vi "RG Configure DAQ auto Max input scale.vi"(4 "input terminal configuration":i32(ring)=10106 items=["default"=-1, "RSE"=10083, "NRSE"=10078, "Differential"=10106, "Pseudodifferential"=12529], 6 "DAQ Card Type":enum16{"USB-6211", "USB-6251", "USB-6361"}(ring)=enum."USB-6251", 7 "Sampling rate":dbl=20000.0, 8 "error in":errorcluster, 9 "DAQ Trigger Level":dbl format="%0.2f", 10 "physical channel":string="Dev2/ai0", 11 "number of samples":i32=100000) -> (0 "error out":errorcluster, 3 "task out":refnum<k21>)   [LabVIEW 2017, in "DAQ.lvlib"]
uses:
  DAQ.lvlib
  <vilib>/DAQmx/read.llb/DAQmx Read (Analog Wfm 1Chan NSamp).vi
  <vilib>/Analysis/baseanly.llb/Mean (DBL).vi
  <vilib>/DAQmx/create/channels.llb/DAQmx Create Channel (AI-Voltage-Basic).vi
  <vilib>/DAQmx/configure/timing.llb/DAQmx Timing (Sample Clock).vi
  <vilib>/DAQmx/miscellaneous.llb/DAQmx Fill In Error Info.vi
  <vilib>/DAQmx/configure/trigger.llb/DAQmx Trigger.vi
  <vilib>/DAQmx/configure/trigger.llb/DAQmx Reference Trigger (Digital Edge).vi
  <vilib>/DAQmx/configure/trigger.llb/DAQmx Reference Trigger (Analog Edge).vi
  <vilib>/Analysis/NI_AALBase.lvlib
  <resource>/objmgr/daqmx.rc
panel:
  out "Input Maximum":dbl format="%#_13g"
  out "pre-trigger samples":u32=10000
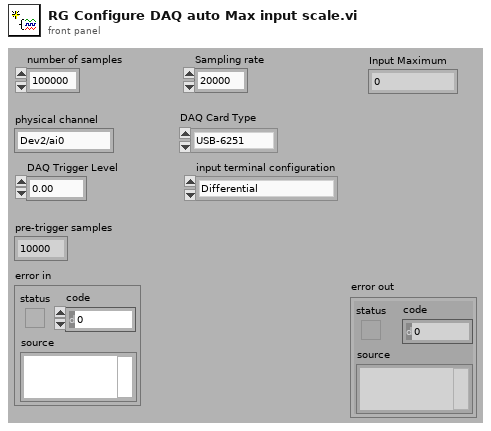
[diagram p1: front panel]
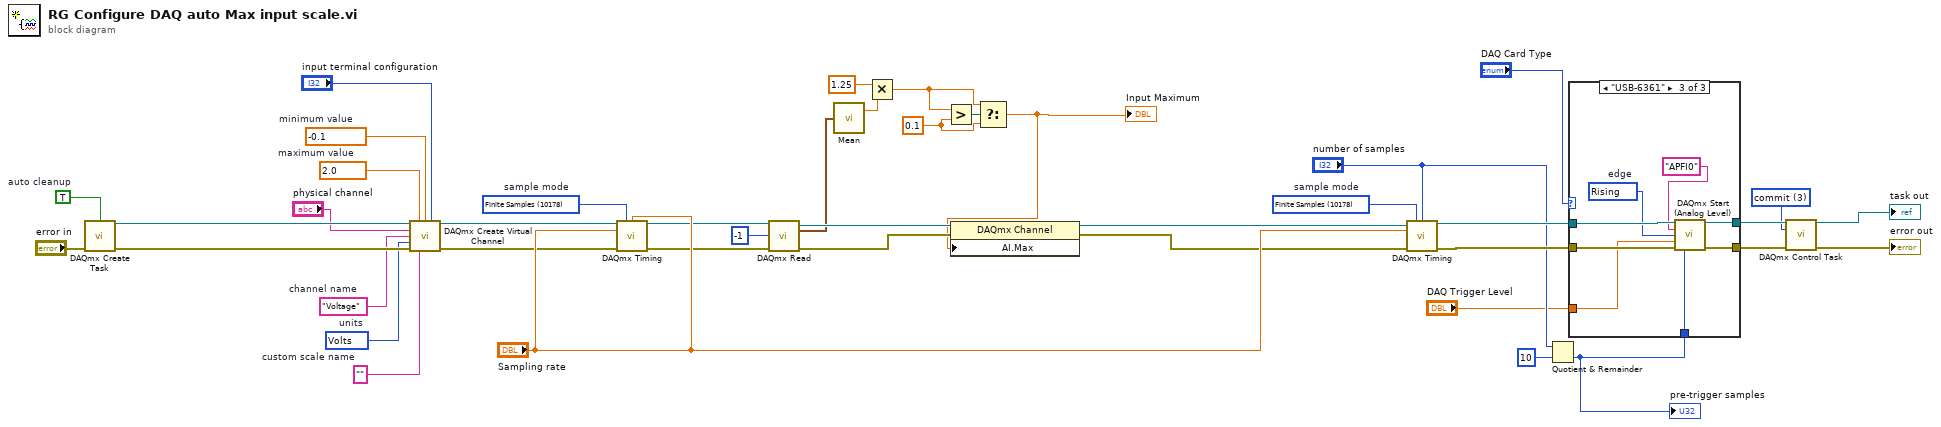
[diagram p0: block diagram]
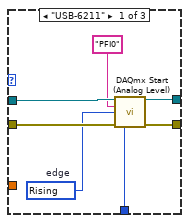
[diagram p2: hidden frame]
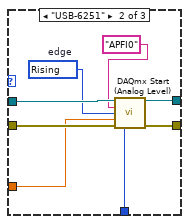
[diagram p3: hidden frame]
diagram:
  w10 = 0.1 ("y")
  w24 = 10178 items=["Finite Samples"=10178, "Continuous Samples"=10123, "Hardware Timed Single Point"=12522]  # sample mode
  w25 = 3 items=["verify"=2, "reserve"=4, "commit"=3, "unreserve"=5, "abort"=6] ("action")
  w35 = 10178 items=["Finite Samples"=10178, "Continuous Samples"=10123, "Hardware Timed Single Point"=12522]  # sample mode
  w15 = 10348 items=["Volts"=10348, "From Custom Scale"=10065]  # units
  w14 = "Voltage"  # channel name
  w37 = ""  # custom scale name
  w13 = -0.1  # minimum value
  w38 = 2.0  # maximum value
  w40 = TRUE  # auto cleanup
  n1 = call <vilib>:"DAQmx Create Task.vi"("auto cleanup"=w40, "error in"="error in") -> ("task out"=w39:refnum<k21>, "error out"=w41:errorcluster)  [unwired: 12 in]
  n2 = call-poly <vilib>:"DAQmx Create Virtual Channel.vi"("task in"=w39, "maximum value"=w38, "minimum value"=w13, "input terminal configuration"="input terminal configuration", "physical channels"="physical channel", "name to assign"=w14, "units"=w15, "error in"=w41, "custom scale name"=w37) -> ("task out"=w21:refnum<k21>, "error out"=w22:errorcluster)  [unwired: 5 in]
  n3 = call-poly <vilib>:"DAQmx Timing.vi"("task/channels in"=w21, "sample mode"=w24, "samples per channel"="Sampling rate", "rate"="Sampling rate", "error in"=w22) -> ("task out"=w20:refnum<k21>, "error out"=w19:errorcluster)  [unwired: 9 in]
  n4 = call-poly <vilib>:"DAQmx Read.vi"("task/channels in"=w20, "number of samples per channel"=-1, "error in"=w19) -> ("task out"=w7:refnum<k21>, "data"=w2:waveform(dbl), "error out"=w6:errorcluster)  [unwired: 10 in]
  n5 = call-poly <vilib>:"Mean.vi"("X"=w2) -> ("mean"=w18:dbl)  [unwired: 1 out]
  n6 = Multiply(x=1.25, y=w18) -> (x*y=w9:dbl)
  n7 = Greater?(x=w9, y=w10) -> (0:w11:bool)
  n8 = Select(t=w9, s=w11, f=w10) -> (s? t:f=w5:dbl)
  "Input Maximum" <- w5
  n9 = property class="DAQmx Channel"(reference=w7, error in=w6, "AI.Max"=w5) -> (reference out=w4:refnum<k21>, error out=w3:errorcluster)
  n10 = call-poly <vilib>:"DAQmx Timing.vi"("task/channels in"=w4, "sample mode"=w35, "samples per channel"="number of samples", "rate"="Sampling rate", "error in"=w3) -> ("task out"=w34:refnum<k21>, "error out"=w36:errorcluster)  [unwired: 9 in]
  n11 = Quotient & Remainder(x="number of samples", y=10) -> (floor(x/y)=w31:i32)  [unwired: 1 out]
  "pre-trigger samples" <- w31
  n12 = case shown="\"USB-6361\"" "DAQ Card Type" {
    tunnel: w36 -> [w49 w57 w65]
    tunnel: [w48 w56 w64] -> w29
    tunnel: [w47 w55 w63] -> w28
    tunnel: w34 -> [w46 w54 w62]
    tunnel: w31 -> [w43 w51 w59]
    tunnel: "DAQ Trigger Level" -> [_ w50 w58]
    frame "USB-6211" {
      w45 = 10280 items=["Rising"=10280, "Falling"=10171]  # edge
      n13 = call-poly "DAQmx Start (Analog Level).vi"("task/channels in"=w46, "source"="PFI0", "edge"=w45, "error in"=w49, "pretrigger samples per channel"=w43) -> ("task out"=w48:refnum<k21>, "error out"=w47:errorcluster)  [unwired: 9 in]
    }
    frame "USB-6251" {
      w53 = 10280 items=["Rising"=10280, "Falling"=10171]  # edge
      n14 = call-poly "DAQmx Start (Analog Level).vi"("task/channels in"=w54, "source"="APFI0", "slope"=w53, "level"=w50, "error in"=w57, "pretrigger samples per channel"=w51) -> ("task out"=w56:refnum<k21>, "error out"=w55:errorcluster)  [unwired: 8 in]
    }
    frame "USB-6361" {
      w61 = 10280 items=["Rising"=10280, "Falling"=10171]  # edge
      n15 = call-poly "DAQmx Start (Analog Level).vi"("task/channels in"=w62, "source"="APFI0", "slope"=w61, "level"=w58, "error in"=w65, "pretrigger samples per channel"=w59) -> ("task out"=w64:refnum<k21>, "error out"=w63:errorcluster)  [unwired: 8 in]
    }
  }
  n16 = call <vilib>:"DAQmx Control Task.vi"("task/channels in"=w29, "action"=w25, "error in"=w28) -> ("task out"=→"task out":refnum<k21>, "error out"=→"error out":errorcluster)  [unwired: 11 in]
